vi "Square Gated IRF Fit Result File String.vi"(8 "error in (no error)":errorcluster, 9 "Square Pulse Statistics":T1 {"Falling Edge Width" format="%0.2f"; "Rising Edge Width" format="%0.2f"; "Falling Edge Midpoint" format="%0.2f"; "Rising Edge Midpoint" format="%0.2f"; "Low Level" format="%0.2f"; "High Level" format="%0.2f"}, 11 "ROI Descriptor":T2 {"Contours"."Type" items=["No Selection", "Point", "Line", "Rectangle", "Oval", "Polygon", "Freehand Region", "Annulus", "Unused2", "Unused3", "Broken Line", "Freehand Line", "Rotated Rectangle"]}) -> (0 "error out":errorcluster, 3 "Result String":string, 5 "Header String":string="ROI_x\tROI_y\tAL\tAL_err\tAU\tAU_err\tx0R\tx0R_err\tdxR\tdxR_err\tx0F\tx0F_err\tdxF\tdxF_err\tR^2\tRMSE\tMethod\tCalls\tIterations")   [LabVIEW 2021, in "Fits.lvlib"]
uses:
  Fits.lvlib
  Square Pulse/Square Pulse Statistics.ctl
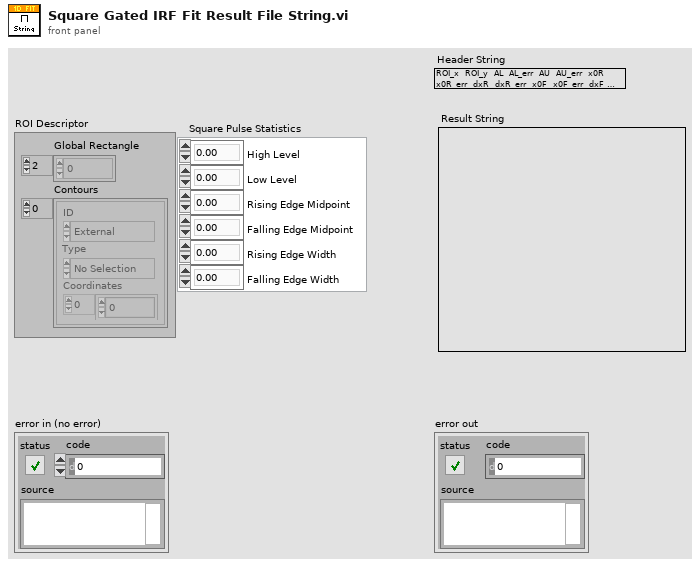
[diagram p1: front panel]
types:
  T1 = typedef "Fits.lvlib/Square Pulse Statistics.ctl" = cluster{"High Level":dbl, "Low Level":dbl, "Rising Edge Midpoint":dbl, "Falling Edge Midpoint":dbl, "Rising Edge Width":dbl, "Falling Edge Width":dbl}
  T2 = typedef "ROI Descriptor" = cluster{"Global Rectangle":i32[], "Contours":cluster{"ID":enum32{"External", "Internal"}, "Type":u32, "Coordinates":i32[]}[]}
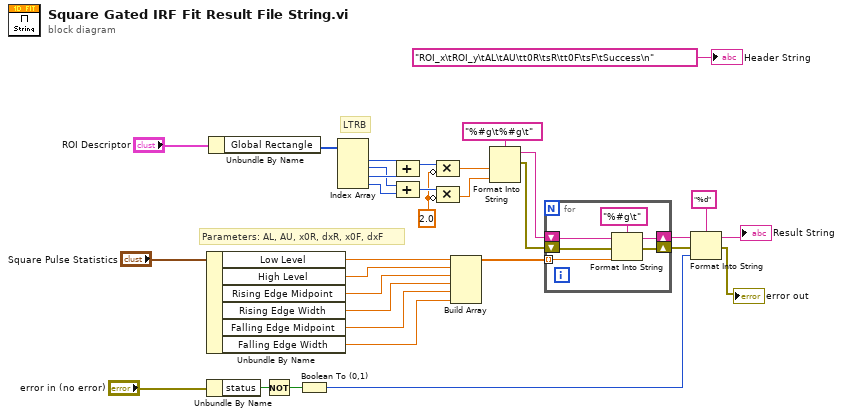
[diagram p0: block diagram]
diagram:
  w17 = 2.0 ("value")
  # "LTRB"
  # "Parameters: AL, AU, x0R, dxR, x0F, dxF"
  n1 = Unbundle By Name("Square Pulse Statistics") -> ("Low Level"=w27:dbl, "High Level"=w13:dbl, "Rising Edge Midpoint"=w12:dbl, "Rising Edge Width"=w11:dbl, "Falling Edge Midpoint"=w10:dbl, "Falling Edge Width"=w9:dbl)
  n2 = Unbundle By Name("error in (no error)") -> ("status"=w3:bool)
  n3 = Unbundle By Name("ROI Descriptor") -> ("Global Rectangle"=w28:i32[])
  n4 = Not(x=w3) -> (.not. x?=w2:bool)
  n5 = Boolean To (0,1)(Boolean=w2) -> (0, 1=w1:i16)
  n6 = Index Array(array=w28) -> (element #1=w26:i32, element #2=w23:i32, element #3=w25:i32, element #4=w24:i32)  [unwired: 4 in]
  n7 = Compound Arithmetic op=ADD(w26, w25) -> (w19:i32)
  n8 = Compound Arithmetic op=ADD(w23, w24) -> (w18:i32)
  n9 = Compound Arithmetic op=MULTIPLY(w19, invert w17) -> (w16:dbl)
  n10 = Compound Arithmetic op=MULTIPLY(w18, invert w17) -> (w15:dbl)
  n11 = Build Array(w27, w13, w12, w11, w10, w9) -> (w14:dbl[])
  n12 = Format Into String(format string="%#g\t%#g\t", w16, w15) -> (resulting string=w20:string, error out=w21:errorcluster)  [unwired: 2 in]
  n13 = for {
    tunnel: w14 -> [w33] mode=indexing
    shift-right: [w36] -> w31
    shift-left: w20 -> [w37]
    shift-right: [w35] -> w7
    shift-left: w21 -> [w34]
    n14 = Format Into String(format string="%#g\t", initial string=w37, error in=w34, w33) -> (resulting string=w36:string, error out=w35:errorcluster)
  }
  n15 = Format Into String(format string="%d", initial string=w31, error in=w7, w1) -> (resulting string=→"Result String":string, error out=→"error out":errorcluster)
  "Header String" <- "ROI_x\tROI_y\tAL\tAU\tt0R\tsR\tt0F\tsF\tSuccess\n" ("format string")
